vi "Init Ring Acquisition.vi"(8 "error in (no error)":errorcluster, 10 "Ring Buffer Size":u32, 11 "Camera Imaqdx in":refnum<class "Camera Imaqdx.lvclass">) -> (0 "error out":errorcluster, 3 "Camera Imaqdx out":refnum<class "Camera Imaqdx.lvclass">)   [LabVIEW 2023, in "Camera Imaqdx.lvclass"]
uses:
  Camera Imaqdx.lvclass
  Camera Imaqdx.lvclass/Camera Imaqdx.ctl
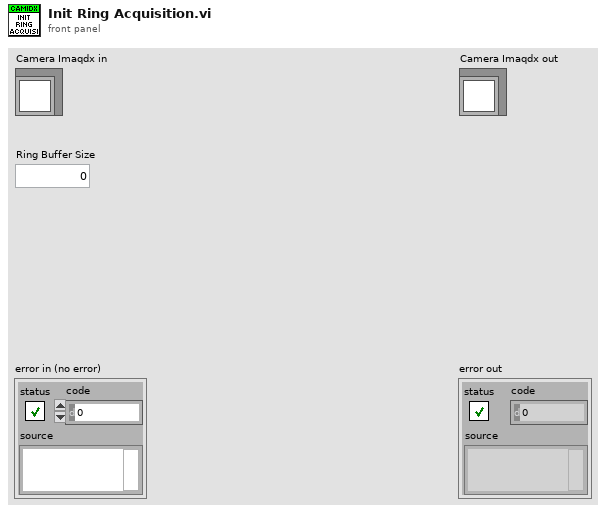
[diagram p1: front panel]
types:
  T1 = typedef "IMAQdx.ctl" = refnum<k21>
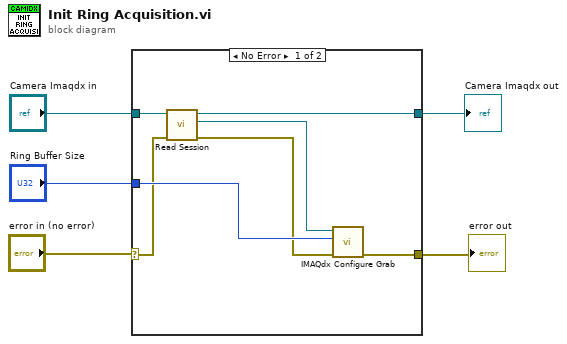
[diagram p0: block diagram]
diagram:
  n1 = case shown="No Error" "error in (no error)" {
    selector: "error in (no error)" -> [w11 w14]
    tunnel: [w10 w14] -> w4
    tunnel: "Camera Imaqdx in" -> [w8 w13]
    tunnel: "Ring Buffer Size" -> [w12 _]
    tunnel: [w7 w13] -> w1
    frame No Error {
      n2 = call "Read Session.vi"("error in (no error)"=w11, "Camera Imaqdx in"=w8) -> ("error out"=w9:errorcluster, "IMAQdx Session"=w6:T1, "Camera Imaqdx out"=w7:refnum<class "Camera Imaqdx.lvclass">)  [unwired: 7 in]
      n3 = call <vilib>:"IMAQdx Configure Grab.vi"("error in"=w9, "Number of Buffers"=w12, "Session In"=w6) -> ("error out"=w10:errorcluster)  [unwired: 7 in, 1 out]
    }
    frame Error {
    }
  }
  "error out" <- w4
  "Camera Imaqdx out" <- w1
